vi "Deploy to Platform.vi"(8 "error in (no error)":errorcluster, 9 "VIA Path":path, 10 "Platform":string, 11 "GVIWebProcessorApp in":refnum<class "GVIWebProcessorApp.lvclass">) -> (0 "error out":errorcluster, 1 "Deployed Resource":string, 2 "Response":string, 3 "GVIWebProcessorApp out":refnum<class "GVIWebProcessorApp.lvclass">)   [LabVIEW 2020, in "PicoG-Processor.lvlib" / "GVIWebProcessorApp.lvclass"]
uses:
  GVIWebProcessorApp.lvclass
  GVIWebProcessorApp.lvclass/GVIWebProcessorApp.ctl
  Builds/picoG/ppl/PicoG-Core.lvlibp/TargetPluginManager/TargetPluginManager.lvclass
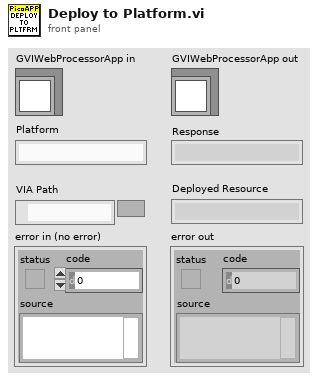
[diagram p1: front panel]
types:
  T1 = enum16{"open", "replace", "create", "open or create", "replace or create", "replace or create with confirmation"}
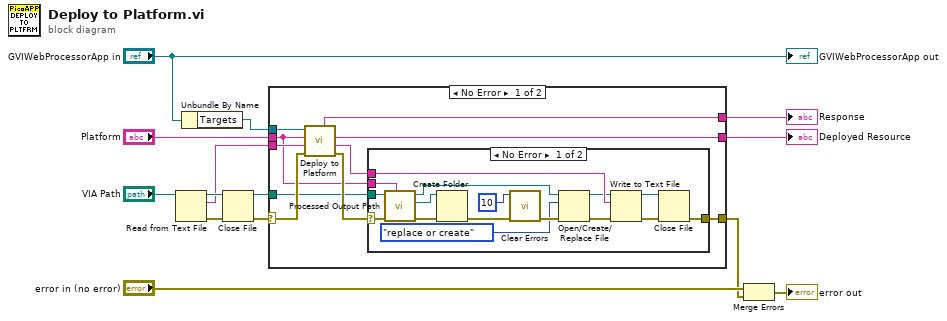
[diagram p0: block diagram]
diagram:
  n1 = Read from Text File(file (use dialog)="VIA Path") -> (refnum out=w12:refnum<file>, text=w2:string, error out=w11:errorcluster)  [unwired: 3 in, 1 out]
  n2 = Unbundle By Name("GVIWebProcessorApp in") -> ("Targets"=w9:refnum<class "TargetPluginManager.lvclass">)
  n3 = Close File(refnum=w12, error in=w11) -> (path=w1:path, error out=w5:errorcluster)
  n4 = case shown="No Error" w5 {
    selector: w5 -> [w20 w41]
    tunnel: w9 -> [w24 _]
    tunnel: "Platform" -> [w15 _]
    tunnel: w2 -> [w23 _]
    tunnel: [w22 _] -> w7
    tunnel: [w21 _] -> w6
    tunnel: [w17 w41] -> w3
    tunnel: w1 -> [w18 _]
    frame No Error {
      n5 = call "Deploy to Platform.vi"("error in (no error)"=w20, "VIA"=w23, "Platform"=w15, "TargetPluginManager in"=w24) -> ("error out"=w19:errorcluster, "Processed VIA"=w16:string, "Deployed Resource"=w21:string, "Response"=w22:string)  [unwired: 3 in, 1 out]
      n6 = case shown="No Error" w19 {
        selector: w19 -> [w36 w40]
        tunnel: w18 -> [w39 _]
        tunnel: [w26 w40] -> w17
        tunnel: w16 -> [w30 _]
        tunnel: w15 -> [w38 _]
        frame No Error {
          n7 = call "Processed Output Path.vi"("Platform"=w38, "Source Via Path"=w39) -> ("Processed Output Folder"=w37:path, "Processed Output Path"=w33:path)  [unwired: 8 in]
          n8 = Create Folder(path (use dialog)=w37, error in=w36) -> (error out=w35:errorcluster)  [unwired: 1 in, 2 out]
          n9 = call <vilib>:"Clear Errors.vi"("error in (no error)"=w35, "specific error code to clear (0: all)"=10) -> ("error out"=w34:errorcluster)  [unwired: 4 in, 1 out]
          n10 = Open/Create/Replace File(file path (use dialog)=w33, error in=w34, operation (0:open)=T1."replace or create") -> (refnum out=w29:refnum<file>, error out=w31:errorcluster)  [unwired: 3 in, 1 out]
          n11 = Write to Text File(file (use dialog)=w29, text=w30, error in=w31) -> (refnum out=w27:refnum<file>, error out=w28:errorcluster)  [unwired: 1 in, 1 out]
          n12 = Close File(refnum=w27, error in=w28) -> (error out=w26:errorcluster)  [unwired: 1 out]
        }
        frame Error {
        }
      }
    }
    frame Error {
    }
  }
  "Response" <- w7
  "Deployed Resource" <- w6
  n13 = Merge Errors("error in (no error)", w3) -> (→"error out":errorcluster)
  "GVIWebProcessorApp out" <- "GVIWebProcessorApp in"
